vi "Self-Test.vi"(8 "error in (no error)":errorcluster, 11 "VISA resource name":refnum<visa-resource-name>) -> (0 "error out":errorcluster, 2 "Result":i16, 3 "VISA resource name out":refnum<visa-resource-name>)   [LabVIEW 2018, in "LTB-1.lvlib" / "3150.lvlib"]
doc: "This VI queries for an internal self-test and places a response into the Output Queue indicating whether or not the device completed the self-test without any detected errors."
uses:
  3150.lvlib
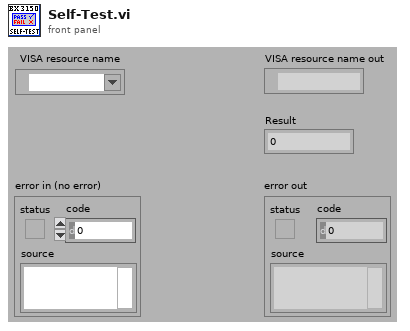
[diagram p1: front panel]
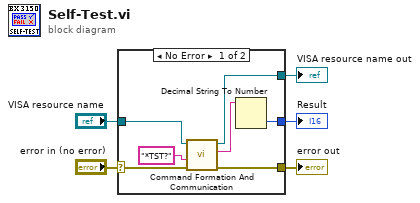
[diagram p0: block diagram]
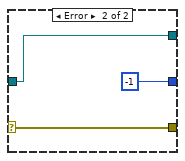
[diagram p2: hidden frame]
diagram:
  n1 = case shown="No Error" "error in (no error)" {
    selector: "error in (no error)" -> [w12 w15]
    tunnel: [w11 w15] -> w1
    tunnel: [w10 w14] -> w3
    tunnel: "VISA resource name" -> [w9 w14]
    tunnel: [w7 -1] -> w5
    frame No Error {
      n2 = call "Command Formation And Communication.vi"("error in (no error)"=w12, "Command"="*TST?", "VISA resource name"=w9) -> ("error out"=w11:errorcluster, "Response"=w6:string, "VISA resource name out"=w10:refnum<visa-resource-name>)  [unwired: 1 in, 5 out]
      n3 = Decimal String To Number(string=w6) -> (number=w7:i32)  [unwired: 3 out]
    }
    frame Error {
    }
  }
  "Result" <- w5
  "VISA resource name out" <- w3
  "error out" <- w1
